vi "configure.vi"(8 "error in (no error)":errorcluster, 9 "Value":i32, 10 "ILC":refnum<class "ILC.lvclass">, 11 "IConfigureILCStrategy in":refnum<class "IConfigureILCStrategy.lvclass">) -> (0 "error out":errorcluster, 3 "IConfigureILCStrategy out":refnum<class "IConfigureILCStrategy.lvclass">)   [LabVIEW 2015, in "IConfigureILCStrategy.lvclass"]
uses:
  IConfigureILCStrategy.lvclass
  <userlib>/Common/ILC/ILC/ILC.lvclass
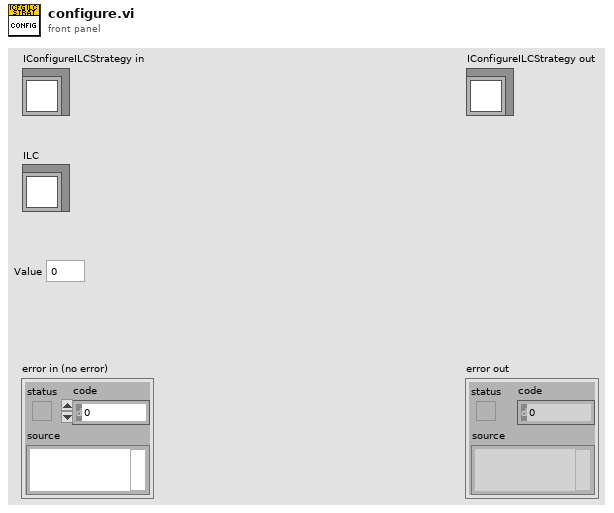
[diagram p1: front panel]
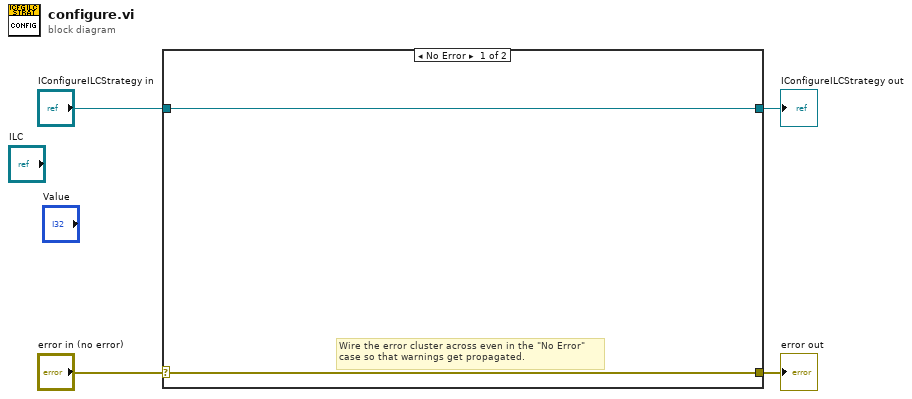
[diagram p0: block diagram]
diagram:
  n1 = case shown="No Error" "error in (no error)" {
    selector: "error in (no error)" -> [w5 w8]
    tunnel: [w5 w8] -> w3
    tunnel: [w6 w7] -> w1
    tunnel: "IConfigureILCStrategy in" -> [w6 w7]
    frame No Error {
      # "Wire the error cluster across even in the \"No Error\"\ncase so that warnings get propagated."
    }
    frame Error {
    }
  }
  "error out" <- w3
  "IConfigureILCStrategy out" <- w1
